vi "Laserdriver_64.vi"() -> ()   [LabVIEW 2022 SP3]
panel:
  out "EnumLasers":string
  out "EnumConnections":string
  out "Numeric":dbl
  in  "OutputPower:":bool
  out "error out":errorcluster
  in  "Laser ON OFF":bool
  in  "Get Status":bool
  in  "Laser Connect":enum32{"Connect", "Disconnect"}(radio)
  in  "Shutter":enum32{"Open", "Atteenuated", "Closed "}(radio)
  out "Status":string[](array[string])
  in  "END":bool
  in  "Set Power:":dbl(slide) scale=0.0..0.30000001192092896
  in  "Communication:":u16(ring) items=["COM1", "COM3", "COM4", "COM6", "COM7", "COM9", "COM10", "COM11", "COM12", "COM13", "LAN10.10.100.120"]
  in  "Lasers":u16(ring) items=["Laser A", "Laser B", "Laser C", "Laser Cx", "Laser D", "Laser Dx", "Laser E"]
  in  "BSALaserCtrl.IBSALaser 2":refnum<k7>
  # "BSA Laser Control Demo"
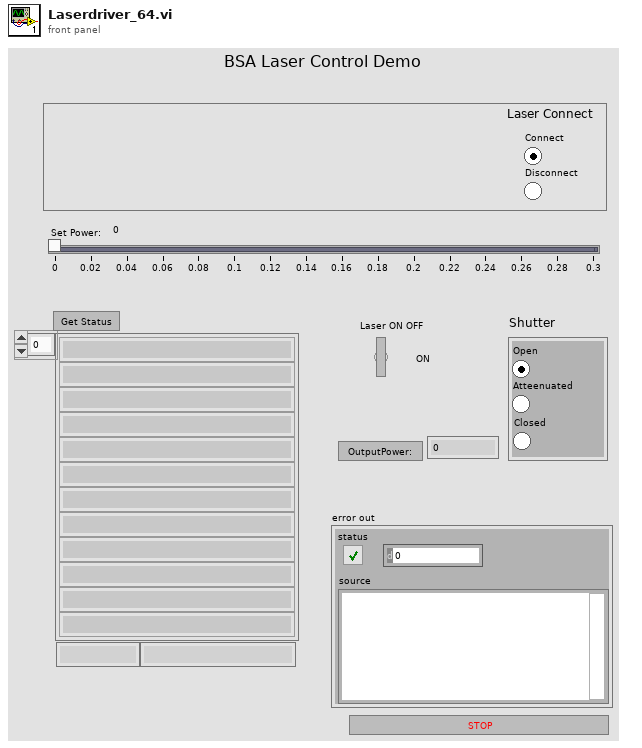
[diagram p1: front panel]
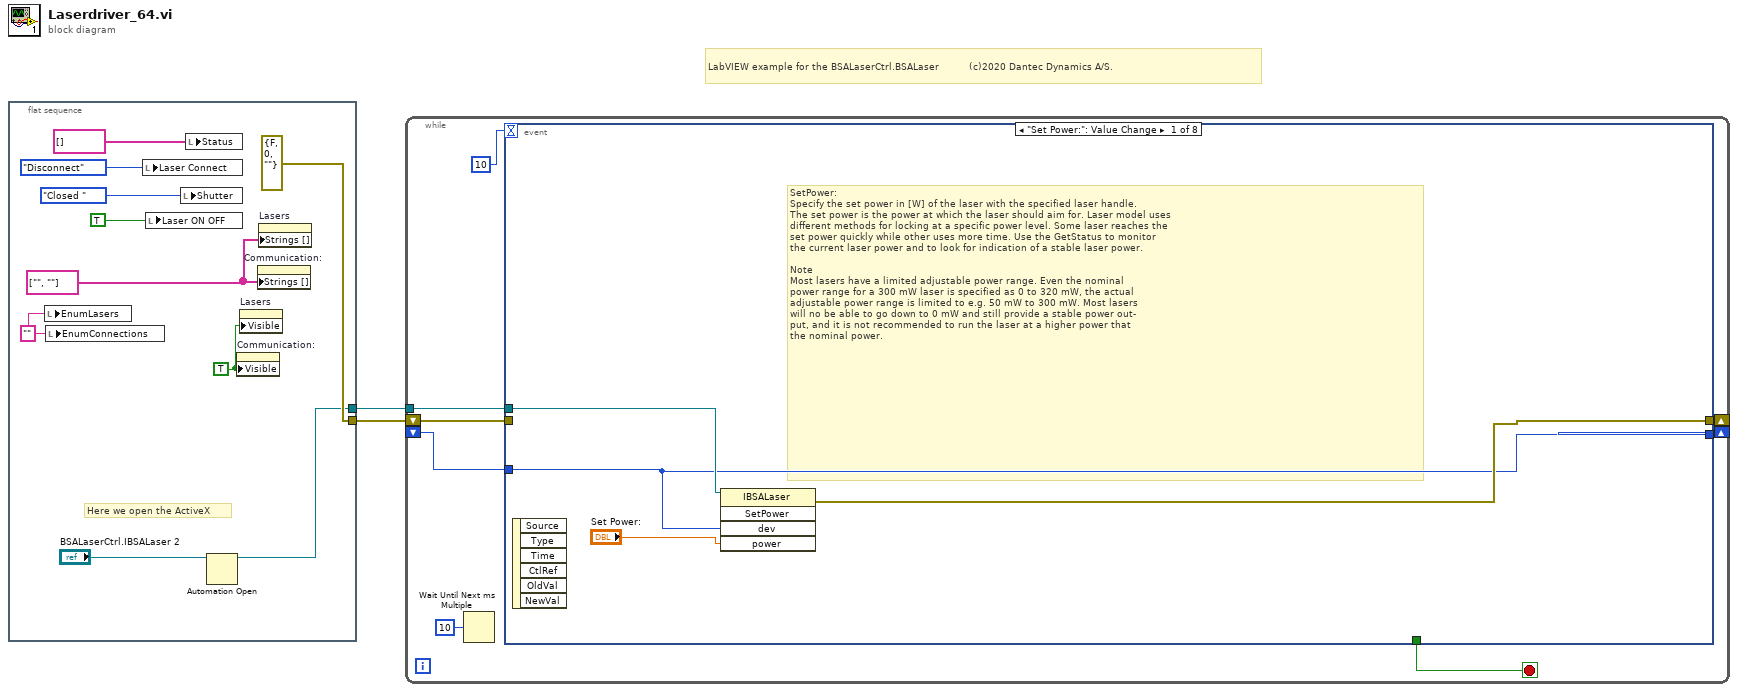
[diagram p0: block diagram]
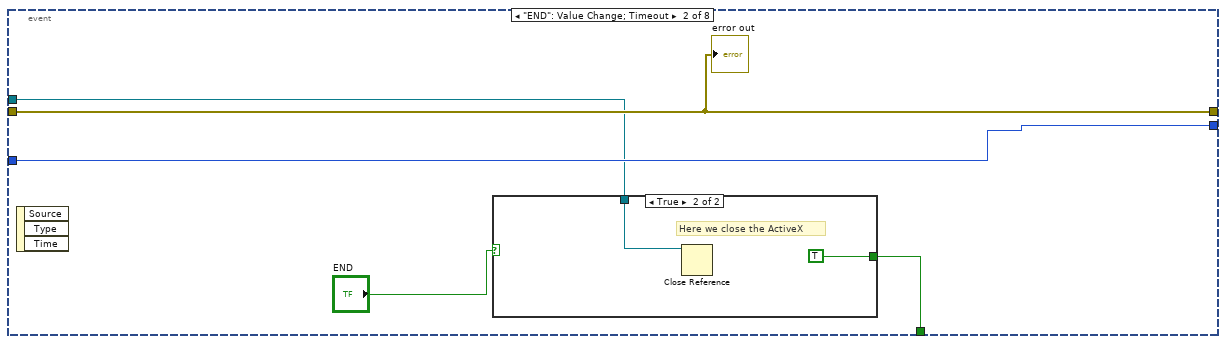
[diagram p2: hidden frame]
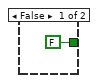
[diagram p3: hidden frame]
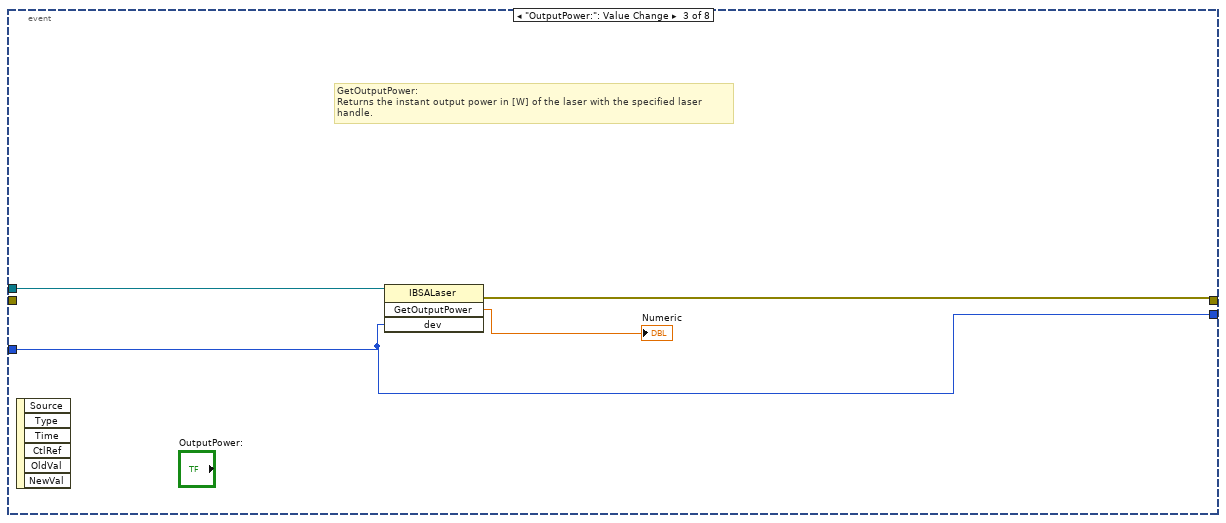
[diagram p4: hidden frame]
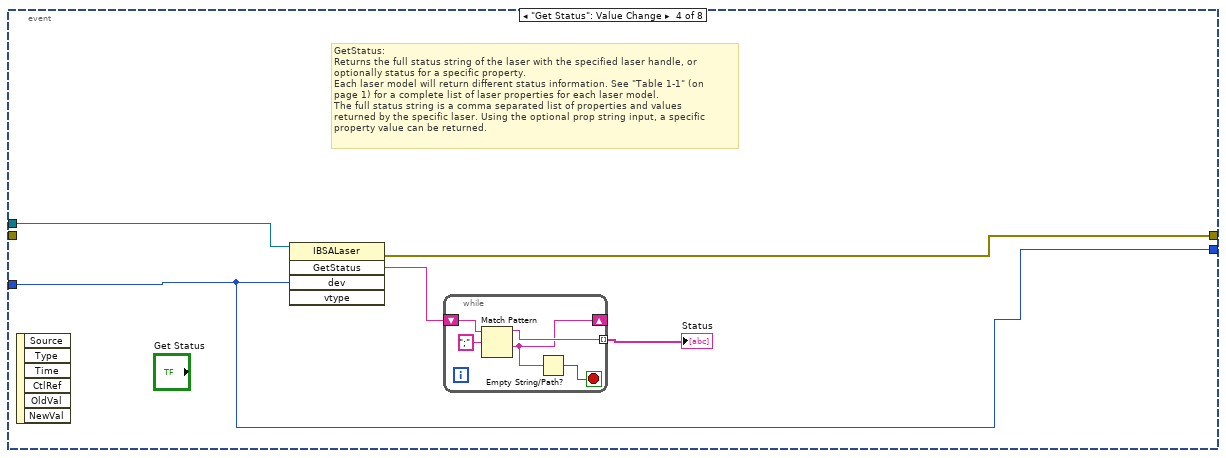
[diagram p5: hidden frame]
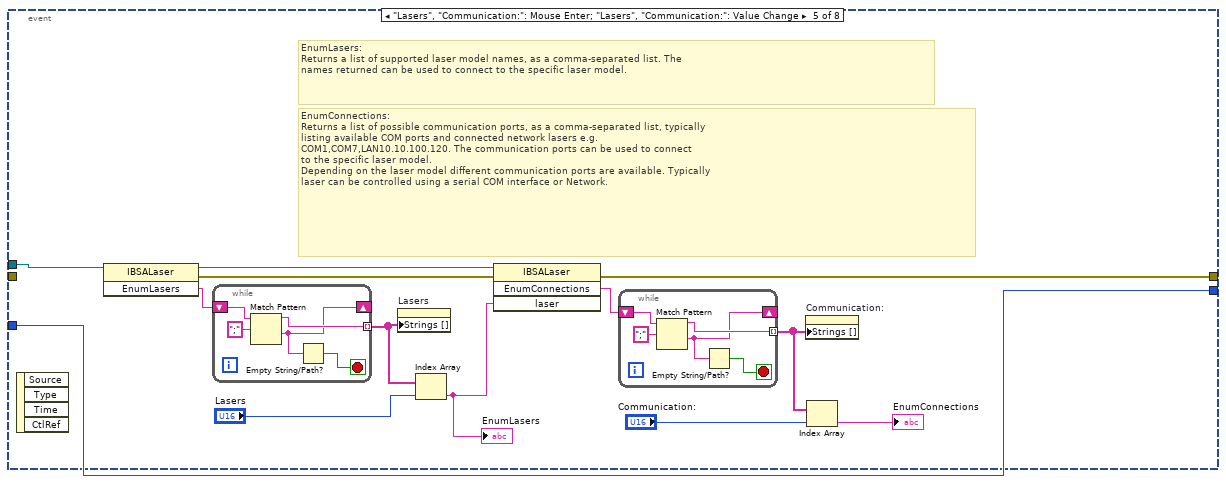
[diagram p6: hidden frame]
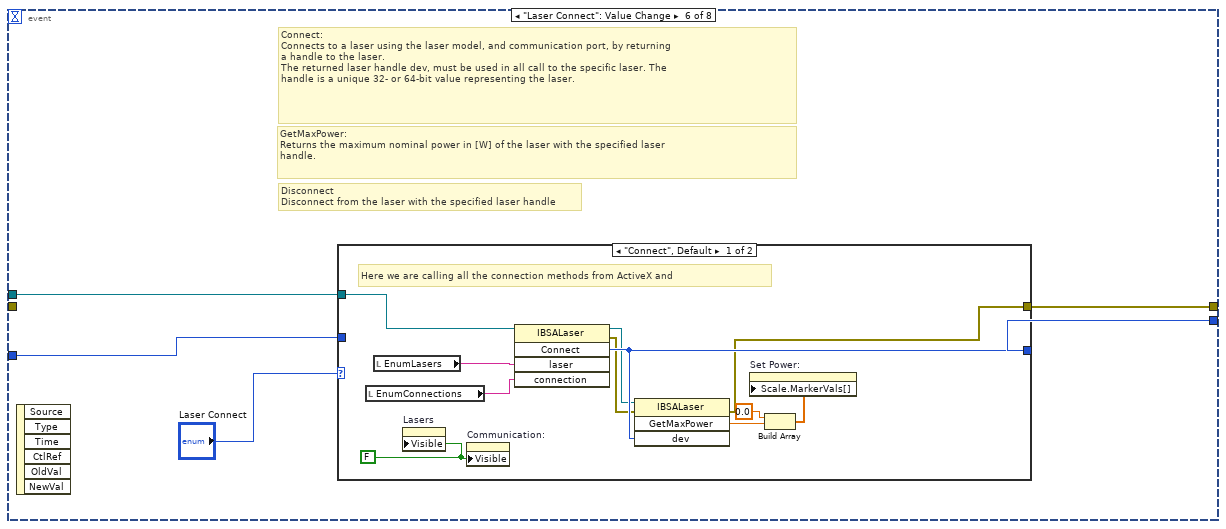
[diagram p7: hidden frame]
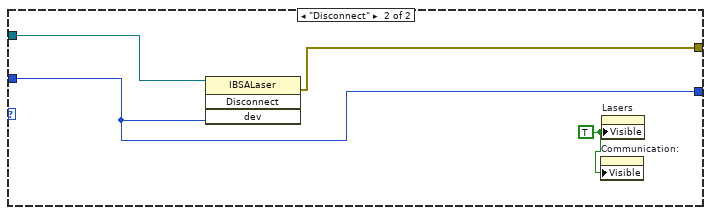
[diagram p8: hidden frame]
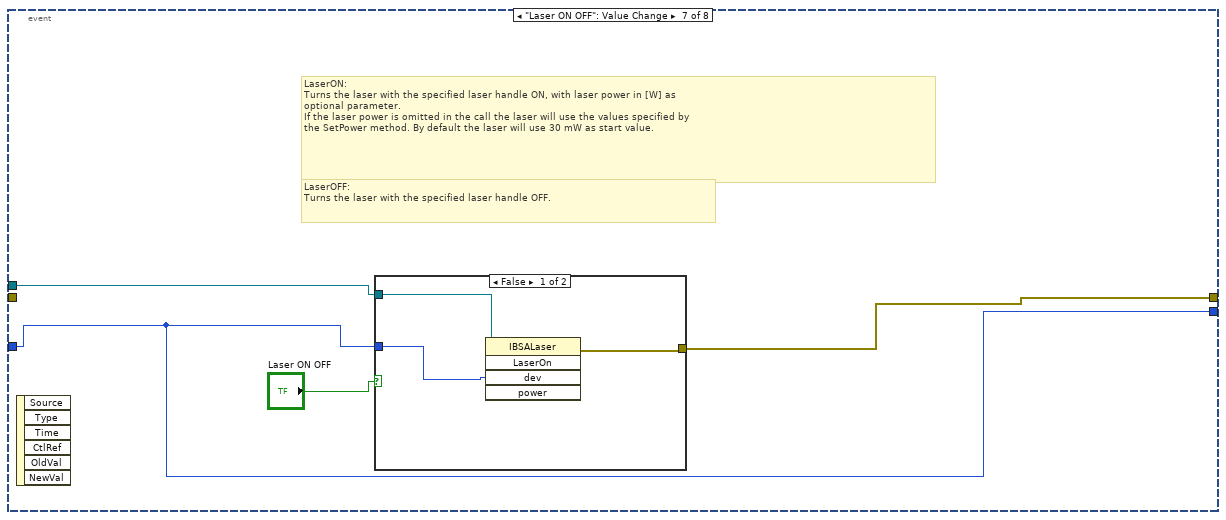
[diagram p9: hidden frame]
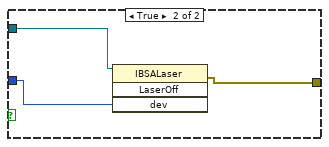
[diagram p10: hidden frame]
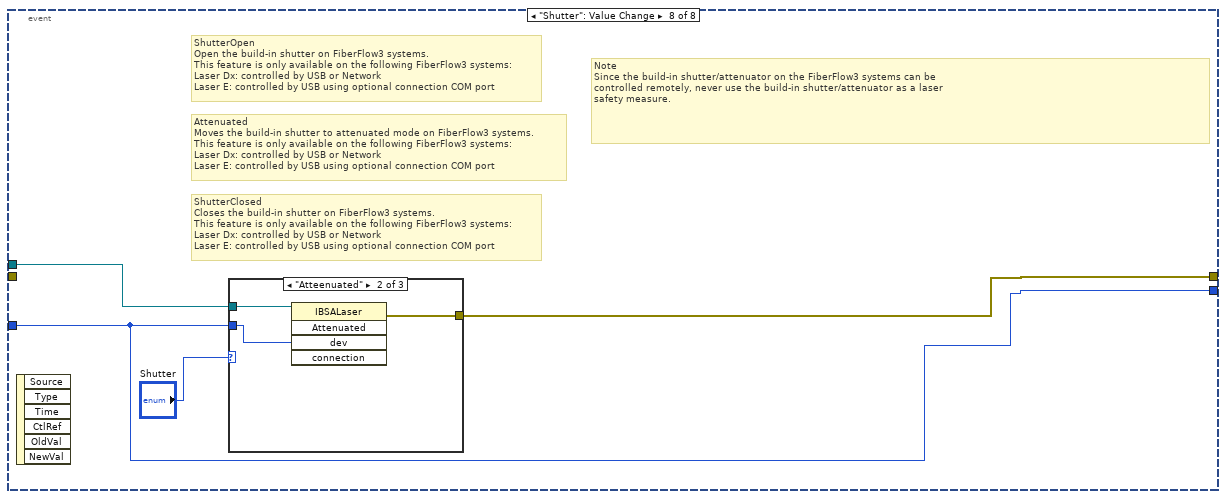
[diagram p11: hidden frame]
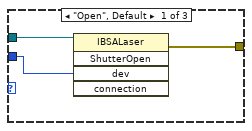
[diagram p12: hidden frame]
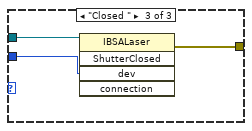
[diagram p13: hidden frame]
diagram:
  # "LabVIEW example for the BSALaserCtrl.BSALaser          (c)2020 Dantec Dynamics A/S."
  n1 = flat-sequence {
    tunnel: [errorcluster {"status"=FALSE, "code"=0, "source"=""} ("error out")] -> w2
    tunnel: [w10] -> w1
    frame #0 {
      w3 = "" ("EnumConnections")
      w4 = TRUE ("Visible")
      w5 = string[] ["", ""] ("Strings []")
      # "Here we open the ActiveX"
      n2 = local write "EnumLasers"(w3) -> ()
      n3 = local write "EnumConnections"(w3) -> ()
      n4 = local write "Laser Connect"(enum32{"Connect", "Disconnect"}."Disconnect" ("Laser Connect")) -> ()
      n5 = local write "Laser ON OFF"(TRUE ("Laser ON OFF")) -> ()
      n6 = local write "Shutter"(enum32{"Open", "Atteenuated", "Closed "}."Closed " ("Shutter")) -> ()
      n7 = local write "Status"(string[] [] ("Status")) -> ()
      n8 = Automation Open(Automation Refnum="BSALaserCtrl.IBSALaser 2") -> (Automation Refnum=w10:refnum<k7>)  [unwired: 3 in, 1 out]
      n9 = property on="Communication:" class="Ring (strict)"("Visible"=w4) -> ()  [unwired: 2 in, 2 out]
      n10 = property on="Lasers" class="Ring (strict)"("Visible"=w4) -> ()  [unwired: 2 in, 2 out]
      n11 = property on="Communication:" class="Ring (strict)"("Strings []"=w5) -> ()  [unwired: 2 in, 2 out]
      n12 = property on="Lasers" class="Ring (strict)"("Strings []"=w5) -> ()  [unwired: 2 in, 2 out]
    }
  }
  n13 = while {
    tunnel: w1 -> [w19]
    shift-right: [w14] -> _
    shift-left: w2 -> [w13]
    shift-right: [w16] -> _
    shift-left: _ -> [w15]
    stop <- w18 stop-if-true
    n14 = Wait Until Next ms Multiple(millisecond multiple=u32 10) -> ()  [unwired: 1 out]
    n15 = event shown="[0] \"Set Power:\": Value Change" {
      selector: _ -> [_ _ _ _ _ _ _ _]
      dyn-events: _ -> [_ _ _ _ _ _ _ _]
      timeout: 10 -> [_ _ _ _ _ _ _ _]
      tunnel: w19 -> [w24 w25 w36 w41 w56 w71 w92 w103]
      tunnel: w15 -> [w21 w29 w34 w39 w53 w72 w90 w100]
      tunnel: [_ w26 _ _ _ _ _ _] -> w18
      tunnel: [w21 w29 w34 w39 w53 w73 w90 w100] -> w16
      tunnel: [w22 w28 w35 w40 w54 w70 w91 w101] -> w14
      tunnel: w13 -> [_ w28 _ _ _ _ _ _]
      event "Set Power:": Value Change {
        # "SetPower:\nSpecify the set power in [W] of the laser with the specified laser handle.\nThe set power is the power at which the laser should aim for. Laser model uses\ndifferent methods for locking at a specific power level. Some laser reaches the\nset power quickly while other uses more time. Use the GetStatus to monitor\nthe current laser power and to look for indication of a stable laser power.\n\nNote\nMost lasers have a limited adjustable power range. Even the nominal\npower range for a 300 mW laser is specified as 0 to 320 mW, the actual\nadjustable power range is limited to e.g. 50 mW to 300 mW. Most lasers\nwill no be able to go down to 0 mW and still provide a stable power out-\nput, and it is not recommended to run the laser at a higher power that\nthe nominal power."
        n16 = event-data() -> ()  [unwired: 1 in, 6 out]
        n17 = invoke class="IBSALaser" method="SetPower"(reference=w24, "dev"=w21, "power"="Set Power:") -> (error out=w22:errorcluster)  [unwired: 2 in, 4 out]
      }
      event "END": Value Change; Timeout {
        n18 = event-data() -> ()  [unwired: 1 in, 3 out]
        n19 = case shown="True" "END" {
          tunnel: [FALSE TRUE] -> w26
          tunnel: w25 -> [_ w31]
          frame False {
          }
          frame True {
            # "Here we close the ActiveX"
            n20 = Close Reference(reference=w31) -> ()  [unwired: 1 in, 1 out]
          }
        }
        "error out" <- w28
      }
      event "OutputPower:": Value Change {
        # "GetOutputPower:\nReturns the instant output power in [W] of the laser with the specified laser\nhandle."
        n21 = event-data() -> ()  [unwired: 1 in, 6 out]
        n22 = invoke class="IBSALaser" method="GetOutputPower"(reference=w36, "dev"=w34) -> (error out=w35:errorcluster, "GetOutputPower"=→"Numeric":dbl)  [unwired: 2 in, 2 out]
      }
      event "Get Status": Value Change {
        # "GetStatus:\nReturns the full status string of the laser with the specified laser handle, or\noptionally status for a specific property.\nEach laser model will return different status information. See \"Table 1-1\" (on\npage 1) for a complete list of laser properties for each laser model.\nThe full status string is a comma separated list of properties and values\nreturned by the specific laser. Using the optional prop string input, a specific\nproperty value can be returned."
        n23 = event-data() -> ()  [unwired: 1 in, 6 out]
        n24 = invoke class="IBSALaser" method="GetStatus"(reference=w41, "dev"=w39) -> (error out=w40:errorcluster, "GetStatus"=w37:string)  [unwired: 3 in, 3 out]
        n25 = while {
          shift-right: [w42] -> _
          shift-left: w37 -> [w45]
          tunnel: [w44] -> w38 mode=indexing
          stop <- w43 stop-if-true
          n26 = Match Pattern(string=w45, regular expression=";") -> (before substring=w44:string, after substring=w42:string)  [unwired: 1 in, 2 out]
          n27 = Empty String/Path?(string/path=w42) -> (empty?=w43:bool)
        }
        "Status" <- w38
      }
      event "Lasers", "Communication:": Mouse Enter; "Lasers", "Communication:": Value Change {
        # "EnumConnections:\nReturns a list of possible communication ports, as a comma-separated list, typically\nlisting available COM ports and connected network lasers e.g.\nCOM1,COM7,LAN10.10.100.120. The communication ports can be used to connect\nto the specific laser model.\nDepending on the laser model different communication ports are available. Typically\nlaser can be controlled using a serial COM interface or Network."
        # "EnumLasers:\nReturns a list of supported laser model names, as a comma-separated list. The\nnames returned can be used to connect to the specific laser model."
        n28 = event-data() -> ()  [unwired: 1 in, 4 out]
        n29 = invoke class="IBSALaser" method="EnumLasers"(reference=w56) -> (reference out=w58:refnum<k7>, error out=w55:errorcluster, "EnumLasers"=w51:string)  [unwired: 2 in]
        n30 = while {
          shift-right: [w65] -> _
          shift-left: w51 -> [w68]
          tunnel: [w67] -> w52 mode=indexing
          stop <- w66 stop-if-true
          n31 = Match Pattern(string=w68, regular expression=";") -> (before substring=w67:string, after substring=w65:string)  [unwired: 1 in, 2 out]
          n32 = Empty String/Path?(string/path=w65) -> (empty?=w66:bool)
        }
        n33 = property on="Lasers" class="Ring (strict)"("Strings []"=w52) -> ()  [unwired: 2 in, 2 out]
        n34 = Index Array(array=w52, index="Lasers") -> (element=w47:string)
        "EnumLasers" <- w47
        n35 = invoke class="IBSALaser" method="EnumConnections"(reference=w58, error in=w55, "laser"=w47) -> (error out=w54:errorcluster, "EnumConnections"=w50:string)  [unwired: 1 in, 2 out]
        n36 = while {
          shift-right: [w60] -> _
          shift-left: w50 -> [w63]
          tunnel: [w62] -> w49 mode=indexing
          stop <- w61 stop-if-true
          n37 = Match Pattern(string=w63, regular expression=";") -> (before substring=w62:string, after substring=w60:string)  [unwired: 1 in, 2 out]
          n38 = Empty String/Path?(string/path=w60) -> (empty?=w61:bool)
        }
        n39 = property on="Communication:" class="Ring (strict)"("Strings []"=w49) -> ()  [unwired: 2 in, 2 out]
        n40 = Index Array(array=w49, index="Communication:") -> (element=→"EnumConnections":string)
      }
      event "Laser Connect": Value Change {
        # "Disconnect\nDisconnect from the laser with the specified laser handle"
        # "GetMaxPower:\nReturns the maximum nominal power in [W] of the laser with the specified laser\nhandle."
        # "Connect:\nConnects to a laser using the laser model, and communication port, by returning\na handle to the laser.\nThe returned laser handle dev, must be used in all call to the specific laser. The\nhandle is a unique 32- or 64-bit value representing the laser."
        n41 = event-data() -> ()  [unwired: 1 in, 6 out]
        n42 = case shown="\"Connect\", Default" "Laser Connect" {
          tunnel: [w82 w88] -> w73
          tunnel: w72 -> [_ w88]
          tunnel: w71 -> [w81 w89]
          tunnel: [w78 w87] -> w70
          frame "Connect", Default {
            w77 = FALSE ("Visible")
            # "Here we are calling all the connection methods from ActiveX and"
            n43 = local read "EnumConnections"() -> (w75:string)
            n44 = local read "EnumLasers"() -> (w76:string)
            n45 = property on="Lasers" class="Ring (strict)"("Visible"=w77) -> ()  [unwired: 2 in, 2 out]
            n46 = property on="Communication:" class="Ring (strict)"("Visible"=w77) -> ()  [unwired: 2 in, 2 out]
            n47 = invoke class="IBSALaser" method="Connect"(reference=w81, "laser"=w76, "connection"=w75) -> (reference out=w80:refnum<k7>, error out=w79:errorcluster, "Connect"=w82:i64)  [unwired: 2 in, 2 out]
            n48 = invoke class="IBSALaser" method="GetMaxPower"(reference=w80, error in=w79, "dev"=w82) -> (error out=w78:errorcluster, "GetMaxPower"=w85:dbl)  [unwired: 1 in, 2 out]
            n49 = Build Array(0.0 ("element"), w85) -> (w84:dbl[])
            n50 = property on="Set Power:" class="Slide (strict)"("Scale.MarkerVals[]"=w84) -> ()  [unwired: 2 in, 2 out]
          }
          frame "Disconnect" {
            w86 = TRUE ("Visible")
            n51 = invoke class="IBSALaser" method="Disconnect"(reference=w89, "dev"=w88) -> (error out=w87:errorcluster)  [unwired: 2 in, 3 out]
            n52 = property on="Communication:" class="Ring (strict)"("Visible"=w86) -> ()  [unwired: 2 in, 2 out]
            n53 = property on="Lasers" class="Ring (strict)"("Visible"=w86) -> ()  [unwired: 2 in, 2 out]
          }
        }
      }
      event "Laser ON OFF": Value Change {
        # "LaserOFF:\nTurns the laser with the specified laser handle OFF."
        # "LaserON:\nTurns the laser with the specified laser handle ON, with laser power in [W] as\noptional parameter.\nIf the laser power is omitted in the call the laser will use the values specified by\nthe SetPower method. By default the laser will use 30 mW as start value."
        n54 = event-data() -> ()  [unwired: 1 in, 6 out]
        n55 = case shown="False" "Laser ON OFF" {
          tunnel: w92 -> [w95 w99]
          tunnel: w90 -> [w96 w98]
          tunnel: [w94 w97] -> w91
          frame False {
            n56 = invoke class="IBSALaser" method="LaserOn"(reference=w95, "dev"=w96) -> (error out=w94:errorcluster)  [unwired: 3 in, 4 out]
          }
          frame True {
            n57 = invoke class="IBSALaser" method="LaserOff"(reference=w99, "dev"=w98) -> (error out=w97:errorcluster)  [unwired: 2 in, 3 out]
          }
        }
      }
      event "Shutter": Value Change {
        # "ShutterClosed\nCloses the build-in shutter on FiberFlow3 systems.\nThis feature is only available on the following FiberFlow3 systems:\nLaser Dx: controlled by USB or Network\nLaser E: controlled by USB using optional connection COM port"
        # "Attenuated\nMoves the build-in shutter to attenuated mode on FiberFlow3 systems.\nThis feature is only available on the following FiberFlow3 systems:\nLaser Dx: controlled by USB or Network\nLaser E: controlled by USB using optional connection COM port"
        # "Note\nSince the build-in shutter/attenuator on the FiberFlow3 systems can be\ncontrolled remotely, never use the build-in shutter/attenuator as a laser\nsafety measure."
        # "ShutterOpen\nOpen the build-in shutter on FiberFlow3 systems.\nThis feature is only available on the following FiberFlow3 systems:\nLaser Dx: controlled by USB or Network\nLaser E: controlled by USB using optional connection COM port"
        n58 = event-data() -> ()  [unwired: 1 in, 6 out]
        n59 = case shown="\"Atteenuated\"" "Shutter" {
          tunnel: w103 -> [w106 w109 w111]
          tunnel: w100 -> [w105 w108 w112]
          tunnel: [w104 w107 w110] -> w101
          frame "Open", Default {
            n60 = invoke class="IBSALaser" method="ShutterOpen"(reference=w106, "dev"=w105) -> (error out=w104:errorcluster)  [unwired: 3 in, 4 out]
          }
          frame "Atteenuated" {
            n61 = invoke class="IBSALaser" method="Attenuated"(reference=w109, "dev"=w108) -> (error out=w107:errorcluster)  [unwired: 3 in, 4 out]
          }
          frame "Closed " {
            n62 = invoke class="IBSALaser" method="ShutterClosed"(reference=w111, "dev"=w112) -> (error out=w110:errorcluster)  [unwired: 3 in, 4 out]
          }
        }
      }
    }
  }
